vi "RichToFlatexternal_driver_wrapper_InitializeRequest.vi"(5 "OutputClusterType":T1, 11 "InputCluster":T2) -> (3 "OutputCluster":T1)   [LabVIEW 2020, in "Instrument Interaction Client.lvlib"]
uses:
  Instrument Interaction Client.lvlib
  external_driver_wrapper_InitializeRequest.ctl
  external_driver_wrapper_InitializeRequest_Flat.ctl
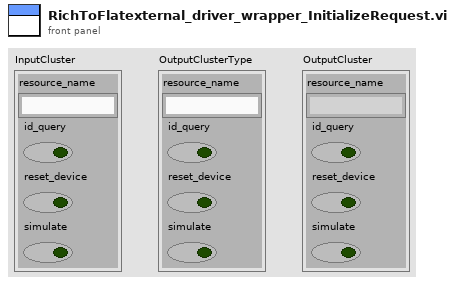
[diagram p1: front panel]
types:
  T1 = typedef "Instrument Interaction Client.lvlib/external_driver_wrapper_InitializeRequest_Flat.ctl" = cluster{"resource_name":string, "id_query":bool, "reset_device":bool, "simulate":bool}
  T2 = typedef "Instrument Interaction Client.lvlib/external_driver_wrapper_InitializeRequest.ctl" = cluster{"resource_name":string, "id_query":bool, "reset_device":bool, "simulate":bool}
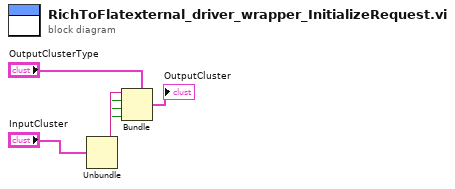
[diagram p0: block diagram]
diagram:
  n1 = Unbundle "Unbundle"("InputCluster") -> ("resource_name"=w4:string, "id_query"=w3:bool, "reset_device"=w2:bool, "simulate"=w1:bool)
  n2 = Bundle "Bundle"(cluster="OutputClusterType", "resource_name"=w4, "id_query"=w3, "reset_device"=w2, "simulate"=w1) -> (→"OutputCluster":T1)
